vi "5.0.5_Inlet_Blockage_Calibration.vi"(6 "Data in":T1, 8 "error in (no error)":errorcluster, 9 "AllControls In":T2, 10 "?":T3, 11 "Message Queue out":T4) -> (0 "error out":errorcluster, 1 "Flow":string, 2 "Data":T3, 3 "Message Queue Out":T4, 4 "Data out":T1)   [LabVIEW 2017]
uses:
  Depends/AMC/subVIs/TypeDefs/amc_Message Queue.ctl
  Depends/AMC/subVIs/TypeDefs/amc_Message.ctl
  Depends/Tools/Keyed Array/Tools_KeyedArray KeyedArray.ctl
  Ctrls/Data.ctl
  Ctrls/AllControls.ctl
  Ctrls/CSV_Data.ctl
  DIPC 692 Daemon API/typdef/get_parameter.ctl
  DIPC 692 Daemon API/typdef/calibration.ctl
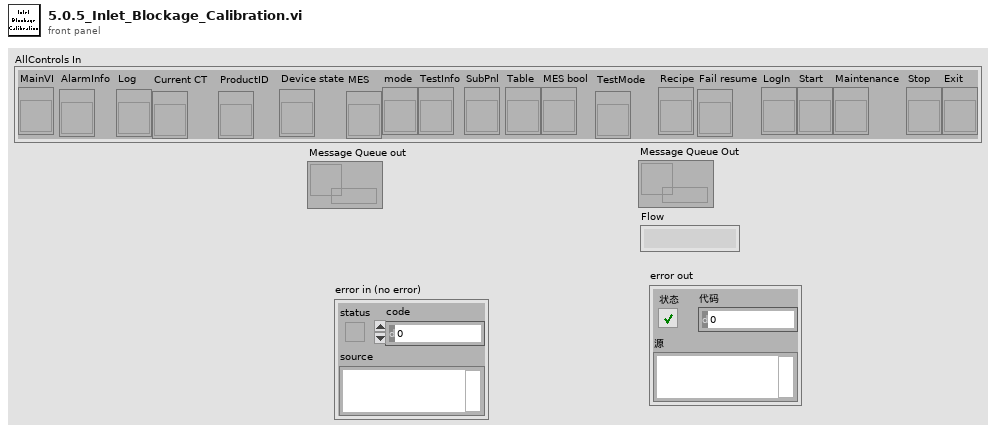
[diagram p1: front panel]
types:
  T1 = typedef "CSV_Data.ctl" = cluster{"Initialisation":cluster{"LMT - Connect UUT (con COM)":string, "LMT - Software Version (rrel)":string, "LMT - Write SKU file (wskuc)":string, "LMT - SKU file name":string, "Connect UUT DDM":string, "Read DDM EOL Timestamp - Mode":string, "Read DDM EOL Timestamp - Timestamp":string, "Read DDM EOL Timestamp - Rig ID":string, "Read DDM EOL Timestamp - Passmark ID":string, "Read DDM EOL Timestamp - Passmark Rev":string, "Software Version before flashing":string, "Read Hardware Serial":string, "UUT DDM SN":string, "Compare DDM SN with MES SN":string, "Backup PCBA Calibration EEPROM Response - CAL":string, "Flash Firmware Version":string, "Check SW Version":string, "Read DDM SW Version after flashing":string, "Set SKU Config":string, "Ready Status":string, "Set Device Mode to EOL":string, "DDM Parameter - Voltage":string, "DDM Parameter - Current":string, "DDM Parameter - Power":string, "DDM Parameter - Speed":string, "DDM Parameter - Pressure":string, "Tester Parameter - Voltage":string, "Tester Parameter - Current":string, "Tester Parameter - Power":string, "Tester Parameter - Ambient Pressure":string, "Tester Parameter - Ambient Temperature":string, "Calculated Parameter - DDM Pressure Corrected":string, "Calculated Parameter - DDM Real Power":string, "Calculated Parameter - Delta V":string}, "BEMF_Calibration":cluster{"Calibration Result - eol_cold_bemf_temp":string, "DDM Ambient Temp":string, "Restriction Plate Diameter":string, "Calibration Result - eol_bemf_mp_cold_coef_a":string, "Calibration Result - eol_bemf_mp_cold_coef_b":string, "Calibration Result - eol_bemf_mp_cold_coef_c":string, "Calibration Result - eol_bemf_lsi_cold_ref_coeffs":string, "Get - Calibration Result - eol_bemf_lsi_speed":string, "Get - Calibration Result - eol_bemf_lsi_integral_0":string, "Calibration Result - eol_bemf_lsi_integral_1":string, "Get - Calibration Result - eol_bemf_lsi_integral_2":string, "Get - Calibration Result - eol_cold_bemf":string, "Get - Calibration Result - eol_cold_bemf_fisf":string, "Finalise Calibration":string, "Compare -Calibration Result - eol_cold_bemf":string, "Compare -Calibration Result - eol_cold_bemf_fisf":string}, "ECO":cluster{"Reset Power Tune":string, "Reset BEMF FISF Calibration":string, "Restriction Plate Diameter":string, "ECO - Stabilisation Time":string, "ECO - DDM Parameter - Voltage":string, "ECO - DDM Parameter - Current":string, "ECO - DDM Parameter - Power":string, "ECO - DDM Parameter - Measured Power":string, "ECO - DDM Parameter - Speed":string, "ECO - DDM Parameter - Pressure":string, "ECO - Tester Parameter - Voltage":string, "ECO - Tester Parameter - Current":string, "ECO - Tester Parameter - Power":string, "ECO - Tester Parameter - Ambient Pressure":string, "ECO - Tester Parameter - Ambient Temperature":string, "ECO - Tester Parameter - Ambient Humidity":string, "ECO - Calculated Parameter - DDM Pressure Corrected":string, "ECO - Calculated Parameter - DDM Real Power":string, "ECO - Calculated Parameter - Delta V":string, "ECO - Calculated Parameter - Flowrate":string, "ECO - Calculated Parameter - Airwatt":string, "ECO - Formula":string, "PT ECO - Power Tune Mode Status":string}, "BOOST":cluster{"Restriction Plate Diameter":string, "BOOST - Stabilisation Time":string, "BOOST - DDM Parameter - Voltage":string, "BOOST - DDM Parameter - Current":string, "BOOST - DDM Parameter - Power":string, "BOOST - DDM Parameter - Measured Power":string, "BOOST - DDM Parameter - Speed":string, "BOOST - DDM Parameter - Pressure":string, "BOOST - Tester Parameter - Voltage":string, "BOOST - Tester Parameter - Current":string, "BOOST - Tester Parameter - Power":string, "BOOST - Tester Parameter - Ambient Pressure":string, "BOOST - Tester Parameter - Ambient Temperature":string, "BOOST - Tester Parameter - Ambient Humidity":string, "BOOST - Calculated Parameter - DDM Pressure Corrected":string, "BOOST - Calculated Parameter - DDM Real Power":string, "BOOST - Calculated Parameter - Delta V":string, "BOOST - Calculated Parameter - Flowrate":string, "BOOST - Calculated Parameter - Airwatt":string, "BOOST - Get AM Presence":string, "Air Muscle Turn Off Status":string, "BOOST - Air Muscle Calculated Parameter - Airwatt B":string, "BOOST - Air Muscle Calculate Airwatt Delta":string, "PT BOOST - Power Tune Mode Status":string, "Finalise Calibration":string, "ECO - Get AW Calibration value":string, "BOOST - Get AW Calibration value":string}, "MAX":cluster{"Restriction Plate Diameter":string, "MAX - Stabilisation Time":string, "Get Average Delta Tmag (LSIdelta_FISFdelta_LSItmag_FISFtmag_IIRtmag)":string, "Get Average Delta Tmag FISF":string, "MAX - DDM Parameter - Voltage":string, "MAX - DDM Parameter - Current":string, "MAX - DDM Parameter - Power":string, "MAX - DDM Parameter - Measured Power":string, "MAX - DDM Parameter - Speed":string, "MAX - DDM Parameter - Pressure":string, "MAX - Tester Parameter - Voltage":string, "MAX - Tester Parameter - Current":string, "MAX - Tester Parameter - Power":string, "MAX - Tester Parameter - Ambient Pressure":string, "MAX - Tester Parameter - Ambient Temperature":string, "MAX - Tester Parameter - Ambient Humidity":string, "MAX - Calculated Parameter - DDM Pressure Corrected":string, "MAX - Calculated Parameter - DDM Real Power":string, "MAX - Calculated Parameter - Delta V":string, "MAX - Calculated Parameter - Flowrate":string, "MAX - Calculated Parameter - Airwatt":string, "MAX_FISF_Check_Average_Delta_Tmag":string, "MAX - FISF - BEMF Finetune Result":string, "MAX tune - Delta P1":string, "MAX tune - Calculated Parameter - Airwatt":string, "Calculate Delta Airwatts - MAX finetune - Delta P2":string, "MAX finetune - DDM Parameter - Voltage":string, "MAX finetune - DDM Parameter - Current":string, "MAX finetune - DDM Parameter - Power":string, "MAX finetune - DDM Parameter - Measured Power":string, "MAX finetune - DDM Parameter - Speed":string, "MAX finetune - DDM Parameter - Pressure":string, "MAX finetune - Tester Parameter - Voltage":string, "MAX finetune - Tester Parameter - Current":string, "MAX finetune - Tester Parameter - Power":string, "MAX finetune - Tester Parameter - Ambient Pressure":string, "MAX finetune - Tester Parameter - Ambient Temperature":string, "MAX finetune - Tester Parameter - Ambient Humidity":string, "MAX finetune - Calculated Parameter - DDM Pressure Corrected":string, "MAX finetune - Calculated Parameter - DDM Real Power":string, "MAX finetune - Calculated Parameter - Delta V":string, "MAX finetune - Calculated Parameter - Flowrate":string, "MAX finetune - Calculated Parameter - Airwatt":string, "Check Derate Result":string, "Delta Tmag FISF":string, "Get Hot BEMF Result":string, "Calculate delta Pressure":string, "Finalise Calibration":string, "Calculate & Check Delta BEMF":string, "Delta P Airwatts Value":string}, "LL":cluster{"DDM Ambient Temp":string, "Restriction Plate Diameter":string, "LL - DDM Parameter - Voltage":string, "LL - DDM Parameter - Current":string, "LL - DDM Parameter - Power":string, "LL - DDM Parameter - Measured Power":string, "LL - DDM Parameter - Speed":string, "LL - DDM Parameter - Pressure":string, "LL - Tester Parameter - Voltage":string, "LL - Tester Parameter - Current":string, "LL - Tester Parameter - Power":string, "LL - DDM Real Power":string, "LL - Calibrate Task Detect LL":string}, "HL":cluster{"HL - DDM Parameter - Voltage":string, "HL - DDM Parameter - Current":string, "HL - DDM Parameter - Power":string, "HL - DDM Parameter - Measured Power":string, "HL - DDM Parameter - Speed":string, "HL - DDM Parameter - Pressure":string, "HL - Tester Parameter - Voltage":string, "HL - Tester Parameter - Current":string, "HL - Tester Parameter - Power":string, "HL - DDM Real Power":string, "HL - Calibrate Task Detect HL":string}, "LH":cluster{"Restriction Plate Diameter":string, "LH - DDM Parameter - Voltage":string, "LH - DDM Parameter - Current":string, "LH - DDM Parameter - Power":string, "LH - DDM Parameter - Measured Power":string, "LH - DDM Parameter - Speed":string, "LH - DDM Parameter - Pressure":string, "LH - Tester Parameter - Voltage":string, "LH - Tester Parameter - Current":string, "LH - Tester Parameter - Power":string, "LH - DDM Real Power":string, "LH - Calibrate Task Detect LH":string}, "HH":cluster{"HH - DDM Parameter - Voltage":string, "HH - DDM Parameter - Current":string, "HH - DDM Parameter - Power":string, "HH - DDM Parameter - Measured Power":string, "HH - DDM Parameter - Speed":string, "HH - DDM Parameter - Pressure":string, "HH - Tester Parameter - Voltage":string, "HH - Tester Parameter - Current":string, "HH - Tester Parameter - Power":string, "HH - DDM Real Power":string, "HH - Calibrate Task Detect HH":string}, "Inlet Blockage Calibration":cluster{"Inlet Blockage Calibration - DDM Parameter - Voltage":string, "Inlet Blockage Calibration - DDM Parameter - Current":string, "Inlet Blockage Calibration - DDM Parameter - Power":string, "Inlet Blockage Calibration - DDM Parameter - Measured Power":string, "Inlet Blockage Calibration - DDM Parameter - Speed":string, "Inlet Blockage Calibration - DDM Parameter - Pressure":string, "Inlet Blockage Calibration - Tester Parameter - Voltage":string, "Inlet Blockage Calibration - Tester Parameter - Current":string, "Inlet Blockage Calibration - Tester Parameter - Power":string, "Inlet Blockage Calibration - DDM Real Power":string, "Calibration Inlet Blockage_E":string, "Finalise Calibration":string, "Get Task Detect LL":string, "Get Task Detect HL":string, "Get Task Detect LH":string, "Get Task Detect HH":string, "Calibration Inlet Blockage":string, "Calibration eol cold bemf temp":string}, "GOOD":cluster{"GOOD UNIT - Clear EEPROM Error Log":string, "GOOD UNIT - Write Product Timestamp - Mode":string, "GOOD UNIT - Write Product Timestamp - Timestamp":string, "GOOD UNIT - Write Product Timestamp - Rig ID":string, "GOOD UNIT - Write Product Timestamp - Passmark ID":string, "GOOD UNIT - Write Product Timestamp - Passmark Rev":string, "GOOD UNIT - Set Device Mode to PROD":string, "GOOD UNIT - Backup PCBA Calibration EEPROM Response":string, "GOOD UNIT - Check Security Bit":string, "GOOD UNIT - Set Calibration Lock":string, "GOOD UNIT - Get_Calibration_Lock":string, "GOOD UNIT - Disconnect UUT":string}, "NG":cluster{"NG UNIT - Read NVM Error":string, "NG UNIT - Set Device Mode to FCT":string, "NG UNIT - Backup PCBA Calibration EEPROM Response - CAL":string, "NG UNIT - Backup PCBA Calibration EEPROM Response - ERROR":string, "NG UNIT - Backup PCBA Calibration EEPROM Response - USAGE":string, "NG UNIT - Disconnect UUT":string}, "SN":string, "Table":string[][], "Count":cluster{"Total":i32, "OK":i32, "NG":i32, "Yield":dbl}, "Start Time":timestamp, "daemon reference":refnum<k5>, "CT":dbl, "Config":string[][], "OK/NG":bool, "Station ID":string, "MES DDM SN":string, "MES PCBA SN":string, "Retest":string, "Lux":string, "Initialisation_Status":cluster{"LMT - Connect UUT (con COM)":string, "LMT - Software Version (rrel)":string, "LMT - Write SKU file (wskuc)":string, "LMT - SKU file name":string, "Connect UUT DDM":string, "Read DDM EOL Timestamp - Mode":string, "Read DDM EOL Timestamp - Timestamp":string, "Read DDM EOL Timestamp - Rig ID":string, "Read DDM EOL Timestamp - Passmark ID":string, "Read DDM EOL Timestamp - Passmark Rev":string, "Software Version before flashing":string, "Read Hardware Serial":string, "UUT DDM SN":string, "Compare DDM SN with MES SN":string, "Backup PCBA Calibration EEPROM Response - CAL":string, "Flash Firmware Version":string, "Check SW Version":string, "Read DDM SW Version after flashing":string, "Set SKU Config":string, "Ready Status":string, "Set Device Mode to EOL":string, "DDM Parameter - Voltage":string, "DDM Parameter - Current":string, "DDM Parameter - Power":string, "DDM Parameter - Speed":string, "DDM Parameter - Pressure":string, "Tester Parameter - Voltage":string, "Tester Parameter - Current":string, "Tester Parameter - Power":string, "Tester Parameter - Ambient Pressure":string, "Tester Parameter - Ambient Temperature":string, "Calculated Parameter - DDM Pressure Corrected":string, "Calculated Parameter - DDM Real Power":string, "Calculated Parameter - Delta V":string}, "BEMF_Calibration_Status":cluster{"Calibration Result - eol_cold_bemf_temp":string, "DDM Ambient Temp":string, "Restriction Plate Diameter":string, "Calibration Result - eol_bemf_mp_cold_coef_a":string, "Calibration Result - eol_bemf_mp_cold_coef_b":string, "Calibration Result - eol_bemf_mp_cold_coef_c":string, "Calibration Result - eol_bemf_lsi_cold_ref_coeffs":string, "Get - Calibration Result - eol_bemf_lsi_speed":string, "Get - Calibration Result - eol_bemf_lsi_integral_0":string, "Calibration Result - eol_bemf_lsi_integral_1":string, "Get - Calibration Result - eol_bemf_lsi_integral_2":string, "Get - Calibration Result - eol_cold_bemf":string, "Get - Calibration Result - eol_cold_bemf_fisf":string, "Finalise Calibration":string, "Compare -Calibration Result - eol_cold_bemf":string, "Compare -Calibration Result - eol_cold_bemf_fisf":string}, "ECO_Status":cluster{"Reset Power Tune":string, "Reset BEMF FISF Calibration":string, "Restriction Plate Diameter":string, "ECO - Stabilisation Time":string, "ECO - DDM Parameter - Voltage":string, "ECO - DDM Parameter - Current":string, "ECO - DDM Parameter - Power":string, "ECO - DDM Parameter - Measured Power":string, "ECO - DDM Parameter - Speed":string, "ECO - DDM Parameter - Pressure":string, "ECO - Tester Parameter - Voltage":string, "ECO - Tester Parameter - Current":string, "ECO - Tester Parameter - Power":string, "ECO - Tester Parameter - Ambient Pressure":string, "ECO - Tester Parameter - Ambient Temperature":string, "ECO - Tester Parameter - Ambient Humidity":string, "ECO - Calculated Parameter - DDM Pressure Corrected":string, "ECO - Calculated Parameter - DDM Real Power":string, "ECO - Calculated Parameter - Delta V":string, "ECO - Calculated Parameter - Flowrate":string, "ECO - Calculated Parameter - Airwatt":string, "ECO - Formula":string, "PT ECO - Power Tune Mode Status":string}, "BOOST_Status":cluster{"Restriction Plate Diameter":string, "BOOST - Stabilisation Time":string, "BOOST - DDM Parameter - Voltage":string, "BOOST - DDM Parameter - Current":string, "BOOST - DDM Parameter - Power":string, "BOOST - DDM Parameter - Measured Power":string, "BOOST - DDM Parameter - Speed":string, "BOOST - DDM Parameter - Pressure":string, "BOOST - Tester Parameter - Voltage":string, "BOOST - Tester Parameter - Current":string, "BOOST - Tester Parameter - Power":string, "BOOST - Tester Parameter - Ambient Pressure":string, "BOOST - Tester Parameter - Ambient Temperature":string, "BOOST - Tester Parameter - Ambient Humidity":string, "BOOST - Calculated Parameter - DDM Pressure Corrected":string, "BOOST - Calculated Parameter - DDM Real Power":string, "BOOST - Calculated Parameter - Delta V":string, "BOOST - Calculated Parameter - Flowrate":string, "BOOST - Calculated Parameter - Airwatt":string, "BOOST - Get AM Presence":string, "Air Muscle Turn Off Status":string, "BOOST - Air Muscle Calculated Parameter - Airwatt B":string, "BOOST - Air Muscle Calculate Airwatt Delta":string, "PT BOOST - Power Tune Mode Status":string, "Finalise Calibration":string, "ECO - Get AW Calibration value":string, "BOOST - Get AW Calibration value":string}, "MAX_Status":cluster{"Restriction Plate Diameter":string, "MAX - Stabilisation Time":string, "Get Average Delta Tmag (LSIdelta_FISFdelta_LSItmag_FISFtmag_IIRtmag)":string, "Get Average Delta Tmag FISF":string, "MAX - DDM Parameter - Voltage":string, "MAX - DDM Parameter - Current":string, "MAX - DDM Parameter - Power":string, "MAX - DDM Parameter - Measured Power":string, "MAX - DDM Parameter - Speed":string, "MAX - DDM Parameter - Pressure":string, "MAX - Tester Parameter - Voltage":string, "MAX - Tester Parameter - Current":string, "MAX - Tester Parameter - Power":string, "MAX - Tester Parameter - Ambient Pressure":string, "MAX - Tester Parameter - Ambient Temperature":string, "MAX - Tester Parameter - Ambient Humidity":string, "MAX - Calculated Parameter - DDM Pressure Corrected":string, "MAX - Calculated Parameter - DDM Real Power":string, "MAX - Calculated Parameter - Delta V":string, "MAX - Calculated Parameter - Flowrate":string, "MAX - Calculated Parameter - Airwatt":string, "MAX_FISF_Check_Average_Delta_Tmag":string, "MAX - FISF - BEMF Finetune Result":string, "MAX tune - Delta P1":string, "MAX tune - Calculated Parameter - Airwatt":string, "Calculate Delta Airwatts - MAX finetune - Delta P2":string, "MAX finetune - DDM Parameter - Voltage":string, "MAX finetune - DDM Parameter - Current":string, "MAX finetune - DDM Parameter - Power":string, "MAX finetune - DDM Parameter - Measured Power":string, "MAX finetune - DDM Parameter - Speed":string, "MAX finetune - DDM Parameter - Pressure":string, "MAX finetune - Tester Parameter - Voltage":string, "MAX finetune - Tester Parameter - Current":string, "MAX finetune - Tester Parameter - Power":string, "MAX finetune - Tester Parameter - Ambient Pressure":string, "MAX finetune - Tester Parameter - Ambient Temperature":string, "MAX finetune - Tester Parameter - Ambient Humidity":string, "MAX finetune - Calculated Parameter - DDM Pressure Corrected":string, "MAX finetune - Calculated Parameter - DDM Real Power":string, "MAX finetune - Calculated Parameter - Delta V":string, "MAX finetune - Calculated Parameter - Flowrate":string, "MAX finetune - Calculated Parameter - Airwatt":string, "Check Derate Result":string, "Delta Tmag FISF":string, "Get Hot BEMF Result":string, "Calculate delta Pressure":string, "Finalise Calibration":string, "Calculate & Check Delta BEMF":string, "Delta P Airwatts Value":string}, "LL_Status":cluster{"DDM Ambient Temp":string, "Restriction Plate Diameter":string, "LL - DDM Parameter - Voltage":string, "LL - DDM Parameter - Current":string, "LL - DDM Parameter - Power":string, "LL - DDM Parameter - Measured Power":string, "LL - DDM Parameter - Speed":string, "LL - DDM Parameter - Pressure":string, "LL - Tester Parameter - Voltage":string, "LL - Tester Parameter - Current":string, "LL - Tester Parameter - Power":string, "LL - DDM Real Power":string, "LL - Calibrate Task Detect LL":string}, "HL_Status":cluster{"HL - DDM Parameter - Voltage":string, "HL - DDM Parameter - Current":string, "HL - DDM Parameter - Power":string, "HL - DDM Parameter - Measured Power":string, "HL - DDM Parameter - Speed":string, "HL - DDM Parameter - Pressure":string, "HL - Tester Parameter - Voltage":string, "HL - Tester Parameter - Current":string, "HL - Tester Parameter - Power":string, "HL - DDM Real Power":string, "HL - Calibrate Task Detect HL":string}, "LH_Status":cluster{"Restriction Plate Diameter":string, "LH - DDM Parameter - Voltage":string, "LH - DDM Parameter - Current":string, "LH - DDM Parameter - Power":string, "LH - DDM Parameter - Measured Power":string, "LH - DDM Parameter - Speed":string, "LH - DDM Parameter - Pressure":string, "LH - Tester Parameter - Voltage":string, "LH - Tester Parameter - Current":string, "LH - Tester Parameter - Power":string, "LH - DDM Real Power":string, "LH - Calibrate Task Detect LH":string}, "HH_Status":cluster{"HH - DDM Parameter - Voltage":string, "HH - DDM Parameter - Current":string, "HH - DDM Parameter - Power":string, "HH - DDM Parameter - Measured Power":string, "HH - DDM Parameter - Speed":string, "HH - DDM Parameter - Pressure":string, "HH - Tester Parameter - Voltage":string, "HH - Tester Parameter - Current":string, "HH - Tester Parameter - Power":string, "HH - DDM Real Power":string, "HH - Calibrate Task Detect HH":string}, "Inlet Blockage Calibration_Status":cluster{"Inlet Blockage Calibration - DDM Parameter - Voltage":string, "Inlet Blockage Calibration - DDM Parameter - Current":string, "Inlet Blockage Calibration - DDM Parameter - Power":string, "Inlet Blockage Calibration - DDM Parameter - Measured Power":string, "Inlet Blockage Calibration - DDM Parameter - Speed":string, "Inlet Blockage Calibration - DDM Parameter - Pressure":string, "Inlet Blockage Calibration - Tester Parameter - Voltage":string, "Inlet Blockage Calibration - Tester Parameter - Current":string, "Inlet Blockage Calibration - Tester Parameter - Power":string, "Inlet Blockage Calibration - DDM Real Power":string, "Calibration Inlet Blockage_E":string, "Finalise Calibration":string, "Get Task Detect LL":string, "Get Task Detect HL":string, "Get Task Detect LH":string, "Get Task Detect HH":string, "Calibration Inlet Blockage":string, "Calibration eol cold bemf temp":string}, "GOOD_Status":cluster{"GOOD UNIT - Clear EEPROM Error Log":string, "GOOD UNIT - Write Product Timestamp - Mode":string, "GOOD UNIT - Write Product Timestamp - Timestamp":string, "GOOD UNIT - Write Product Timestamp - Rig ID":string, "GOOD UNIT - Write Product Timestamp - Passmark ID":string, "GOOD UNIT - Write Product Timestamp - Passmark Rev":string, "GOOD UNIT - Set Device Mode to PROD":string, "GOOD UNIT - Backup PCBA Calibration EEPROM Response":string, "GOOD UNIT - Check Security Bit":string, "GOOD UNIT - Set Calibration Lock":string, "GOOD UNIT - Get_Calibration_Lock":string, "GOOD UNIT - Disconnect UUT":string}, "NG_Status":cluster{"NG UNIT - Read NVM Error":string, "NG UNIT - Set Device Mode to FCT":string, "NG UNIT - Backup PCBA Calibration EEPROM Response - CAL":string, "NG UNIT - Backup PCBA Calibration EEPROM Response - ERROR":string, "NG UNIT - Backup PCBA Calibration EEPROM Response - USAGE":string, "NG UNIT - Disconnect UUT":string}, "SKU":string, "Plate_Diameter":string, "Alarm":string}
  T2 = typedef "AllControls.ctl" = cluster{"MainVI":refnum<vi>, "AlarmInfo":refnum<vi>, "Log":refnum<vi>, "Current CT":refnum<vi>, "ProductID":refnum<vi>, "Device state":refnum<vi>, "MES":refnum<vi>, "mode":refnum<vi>, "TestInfo":refnum<vi>, "SubPnl":refnum<vi>, "Table":refnum<vi>, "MES bool":refnum<vi>, "TestMode":refnum<vi>, "Recipe":refnum<vi>, "Fail resume":refnum<vi>, "LogIn":refnum<vi>, "Start":refnum<vi>, "Maintenance":refnum<vi>, "Stop":refnum<vi>, "Exit":refnum<vi>}
  T3 = typedef "Data.ctl" = cluster{"Initialisation":cluster{"DDM_Parameter":dbl[], "DDM_Parameter_status":bool[], "Get_Tester_Parameter":dbl[], "Get_Tester_Parameter_status":bool[], "Cal_Tester_Parameter":dbl[], "Cal_Tester_Parameter_status":bool[], "sw_version_before_status":bool, "sw_version_after_status":bool, "Set_SKU_Config_With_LMT_status":bool, "FCT_timestamp_status":bool, "LMT_Connect_to_UUT_status":bool}, "BEMF_Calibration":cluster{"Read_ambient_temperature":dbl, "Calibration_Vaule":dbl[], "Calibration_Vaule _B":dbl[], "Calibration_Vaule_status":bool[], "Calibration_Vaule_B_status":bool[]}, "ECO":cluster{"DDM_Parameter":dbl[], "DDM_Parameter_status":bool[], "Get_Tester_Parameter":dbl[], "Get_Tester_Parameter_status":bool[], "Cal_Tester_Parameter":dbl[], "Cal_Tester_Parameter_status":bool[], "DDM_Parameter_after_power_tune":dbl[], "Get_Tester_Parameter_after_power_tune":dbl[], "Cal_Tester_Parameter_after_power_tune":dbl[], "Cal_Tester_Parameter_after_power_tune_status":bool[], "Delta_P":dbl}, "BOOST":cluster{"DDM_Parameter":dbl[], "DDM_Parameter_status":bool[], "Get_Tester_Parameter":dbl[], "Get_Tester_Parameter_status":bool[], "Cal_Tester_Parameter":dbl[], "Cal_Tester_Parameter_status":bool[], "DDM_Parameter_after_power_tune":dbl[], "Get_Tester_Parameter_after_power_tune":dbl[], "Cal_Tester_Parameter_after_power_tune":dbl[], "Cal_Tester_Parameter_after_power_tune_status":bool[], "airwatts_am_off":dbl, "AW_Delta_(AM_on_and_off)":dbl, "AW_Delta_(AM_on_and_off)_Status":bool, "Delta_P":dbl}, "MAX":cluster{"Average_Tmag_Data":cluster{"LSI Delta in degC":dbl, "FISF Delta in degc":dbl, "LSI Tmag in degC":dbl, "Fisf Tmag in degC":dbl, "IIR Tmag in degC":dbl}, "DDM_Parameter":dbl[], "DDM_Parameter_status":bool[], "Get_Tester_Parameter":dbl[], "Get_Tester_Parameter_status":bool[], "Cal_Tester_Parameter":dbl[], "BEMF_Finetune":cluster{"eol_bemf_mp_cold_coef_c":dbl, "eol_cold_bemf_fisf_offset":dbl}, "AW_Tune":cluster{"delta_P1":dbl, "delta_P_Setting":dbl}, "DDM_Parameter_after_Airwatts_Tune":dbl[], "Get_Tester_Parameter_after_Airwatts_Tune":dbl[], "Cal_Tester_Parameter_after_Airwatts_Tune":dbl[], "DDM_Parameter_after_Airwatts_Finetune":dbl[], "Get_Tester_Parameter_after_Airwatts_Finetune":dbl[], "Cal_Tester_Parameter_after_Airwatts_Finetune":dbl[], "AW_Finetune":cluster{"delta_P2":dbl, "delta_P_Setting":dbl}, "Delta_Tmag_after_tune":cluster{"LSI Delta in degC":dbl, "FISF Delta in degc":dbl, "LSI Tmag in degC":dbl, "Fisf Tmag in degC":dbl, "IIR Tmag in degC":dbl}, "Hot Bemf in mV":dbl, "DDM_Pressure":dbl, "Delta_Pressure":dbl, " Cold Bemf in mV":dbl, " delta Bemf":dbl, " delta p":dbl, "Delta_Pressure_status":bool, " delta Bemf_status":bool, "LSI Delta in degC_status":bool, "FISF Delta in degc_status":bool, "Max_check_derate_status_status":bool, "Average_All_data":dbl[][], "Average_Tmag_Data_status":bool[], "Average_Tmag_Data_after_tune_status":bool[], "Cal_Tester_Parameter_status":bool[], "Cal_Tester_Parameter_status_after_Airwatts_Tune":bool[], "Cal_Tester_Parameter_status_after_Airwatts_FineTune":bool[]}, "Task_Detect_Calib":cluster{"LL":cluster{"DDM_Parameter":dbl[], "DDM_Parameter_status":bool[], "Get_Tester_Parameter":dbl[], "Get_Tester_Parameter_status":bool[], "Set_task_detect_A":dbl, "Set_task_detect_A_Status":bool}, "HL":cluster{"DDM_Parameter":dbl[], "DDM_Parameter_status":bool[], "Get_Tester_Parameter":dbl[], "Get_Tester_Parameter_status":bool[], "Set_task_detect_B":dbl, "Set_task_detect_B_Status":bool}, "LH":cluster{"DDM_Parameter":dbl[], "DDM_Parameter_status":bool[], "Get_Tester_Parameter":dbl[], "Get_Tester_Parameter_status":bool[], "Set_task_detect_C":dbl, "Set_task_detect_C_Status":bool}, "HH":cluster{"DDM_Parameter":dbl[], "DDM_Parameter_status":bool[], "Get_Tester_Parameter":dbl[], "Get_Tester_Parameter_status":bool[], "Set_task_detect_D":dbl, "Read_and_check_calibration_Status":bool[], "Set_task_detect_D_Status":bool}, "Get_eol_inlet_blockage_E":dbl, "Calib_vaule":cluster{"Get_task_detect_LL":dbl, "Get_task_detect_HL":dbl, "Get_task_detect_LH":dbl, "Get_task_detect_HH":dbl, "eol_inlet_blockage":dbl, "eol_code_bemf_temp":dbl}, "calibrated temp":dbl, "Inlet_Blockage_Calibration":cluster{"DDM_Parameter":dbl[], "DDM_Parameter_status":bool[], "Get_Tester_Parameter":dbl[], "Get_Tester_Parameter_status":bool[]}, "Get_eol_inlet_blockage_E_Status":bool}, "good":cluster{"Write_Product_TS":cluster{"TIMESTAMP":i64, "RIG_ID":i64, "PASSMARK_ID":i64, "PASSMARK_REV":i64}, "Read_Product_TS":cluster{"TIMESTAMP":i64, "RIG_ID":i64, "PASSMARK_ID":i64, "PASSMARK_REV":i64}, "Good_Check_Secuity_Bit_Stauts":bool}}
  T4 = typedef "amc_Message Queue.ctl" = refnum<queue>
  T5 = typedef "HD Config.ctl" = cluster{" PC":cluster{"PC Address":u8[], "PC Port":i32}, "FCO":cluster{"COM":refnum<visa-resource-name>, "Baudrate":u32}, "DC Power ":cluster{"COM":refnum<visa-resource-name>, "Baudrate":u32}, "PW3336":cluster{"COM":refnum<visa-resource-name>, "Baudrate":u32}, "Lefoo":cluster{"COM":refnum<visa-resource-name>, "Baudrate":u32}, "Tempt&Hum":cluster{"COM":refnum<visa-resource-name>, "Baudrate":u32}, "DIPC":cluster{"COM":refnum<visa-resource-name>}, "Daemon":cluster{"IP Address":string, "Port":u16, "Retry":u16}, "URAT":cluster{"COM":refnum<visa-resource-name>, "Baudrate":u32}, "Fail_resume_mode":bool, "GRR":bool}
  T6 = typedef "get_parameter.ctl" = string
  T7 = typedef "calibration.ctl" = string
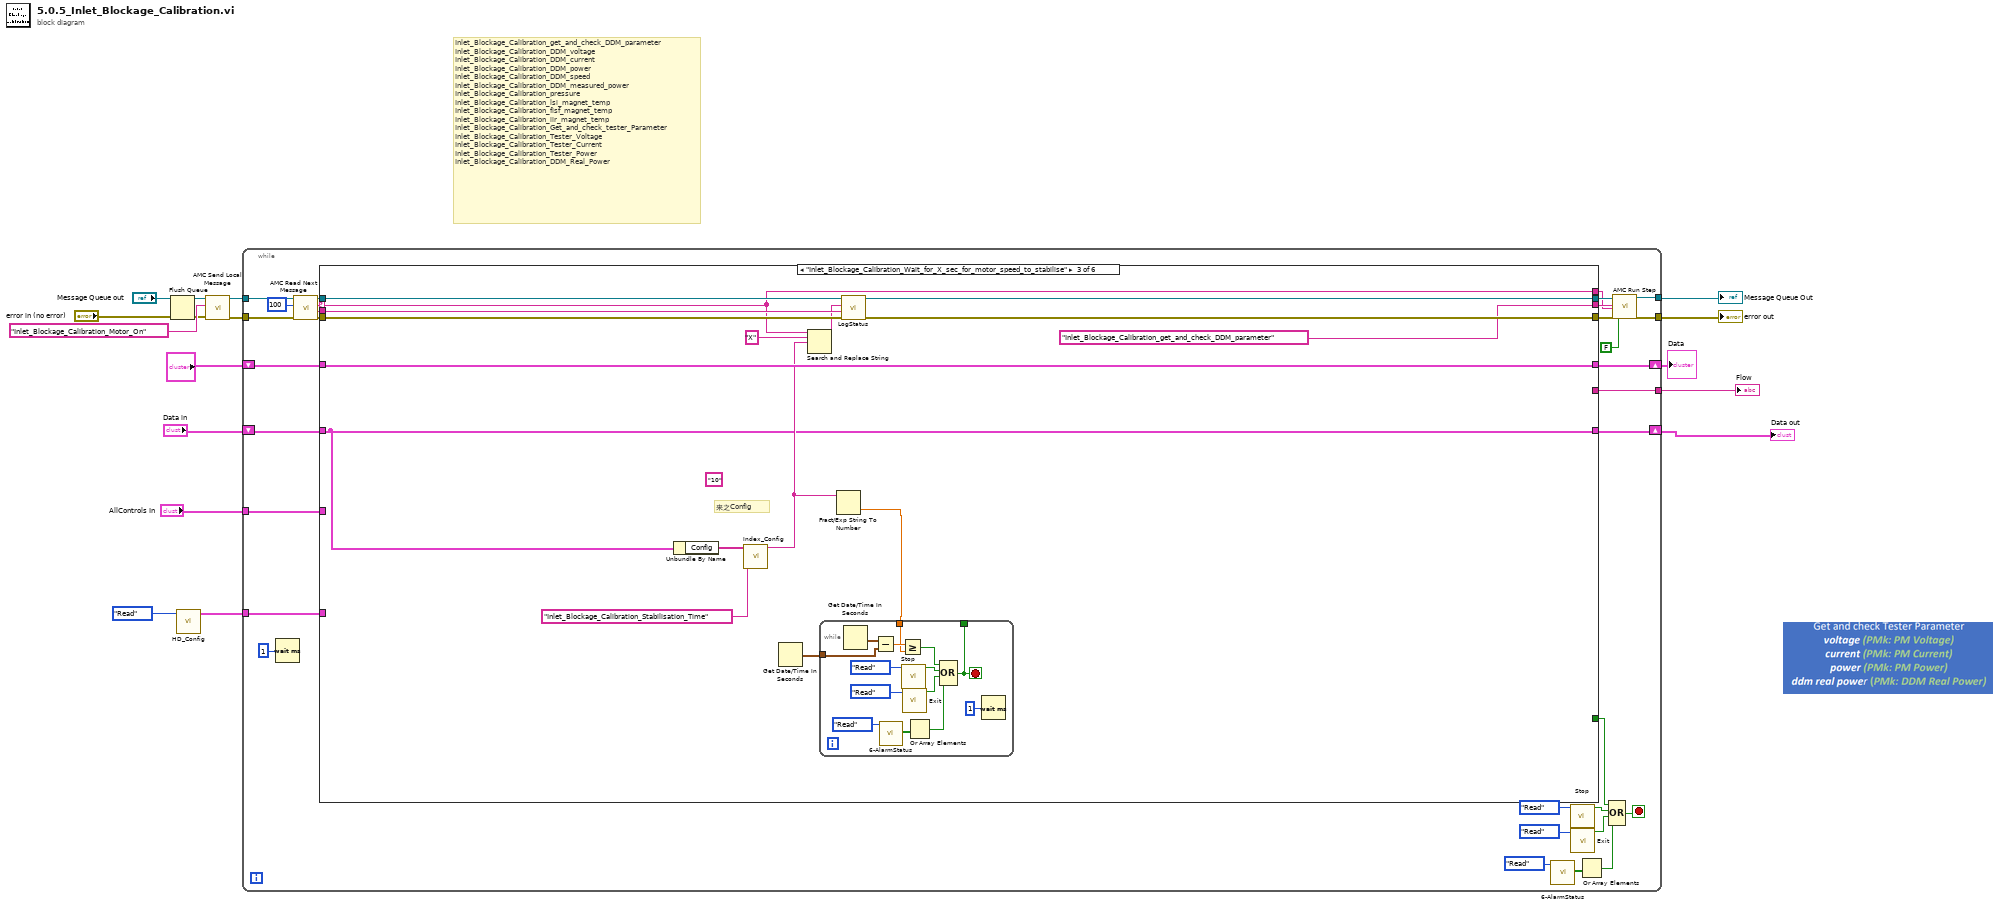
[diagram p0: block diagram]
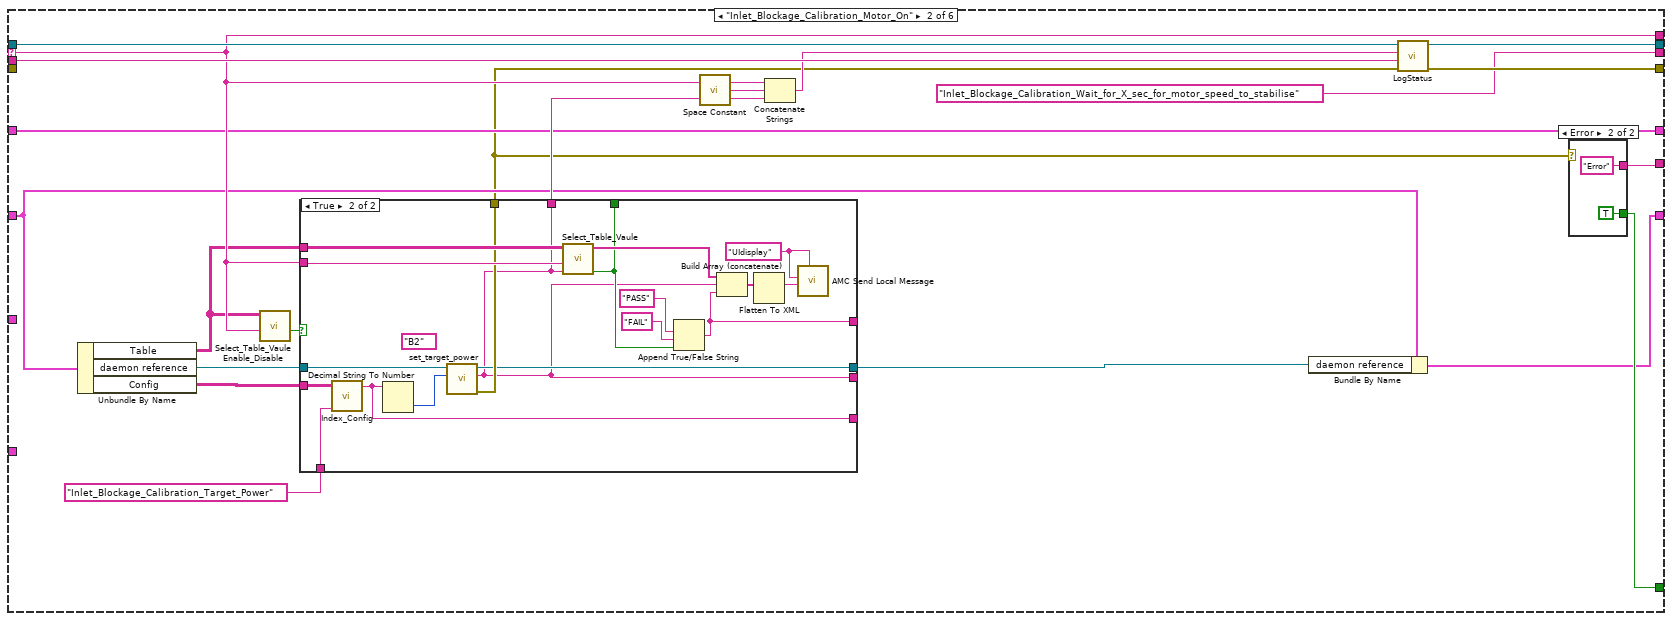
[diagram p3: hidden frame]
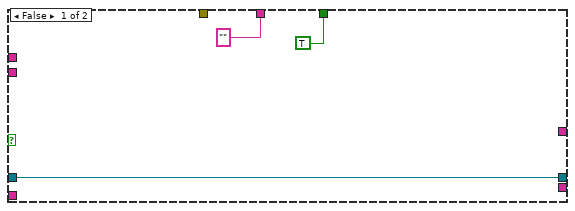
[diagram p5: hidden frame]
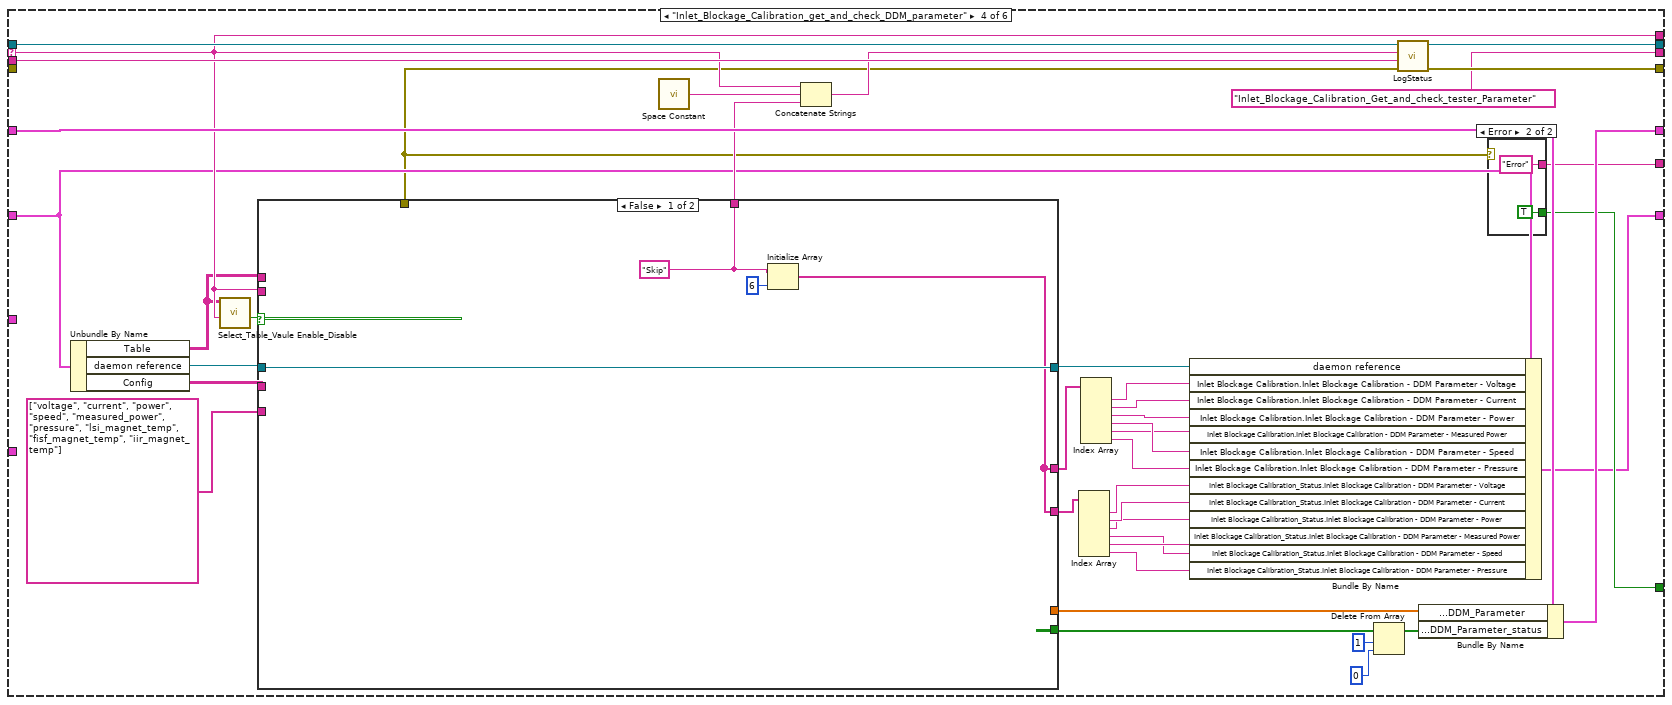
[diagram p6: hidden frame]
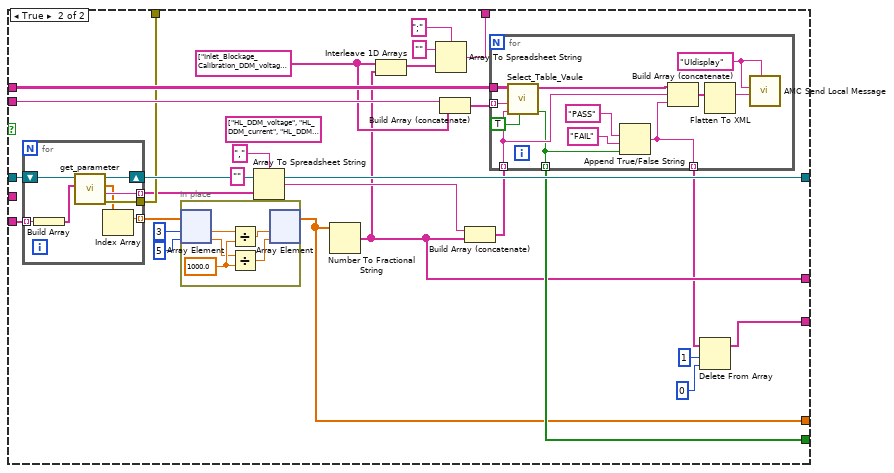
[diagram p8: hidden frame]
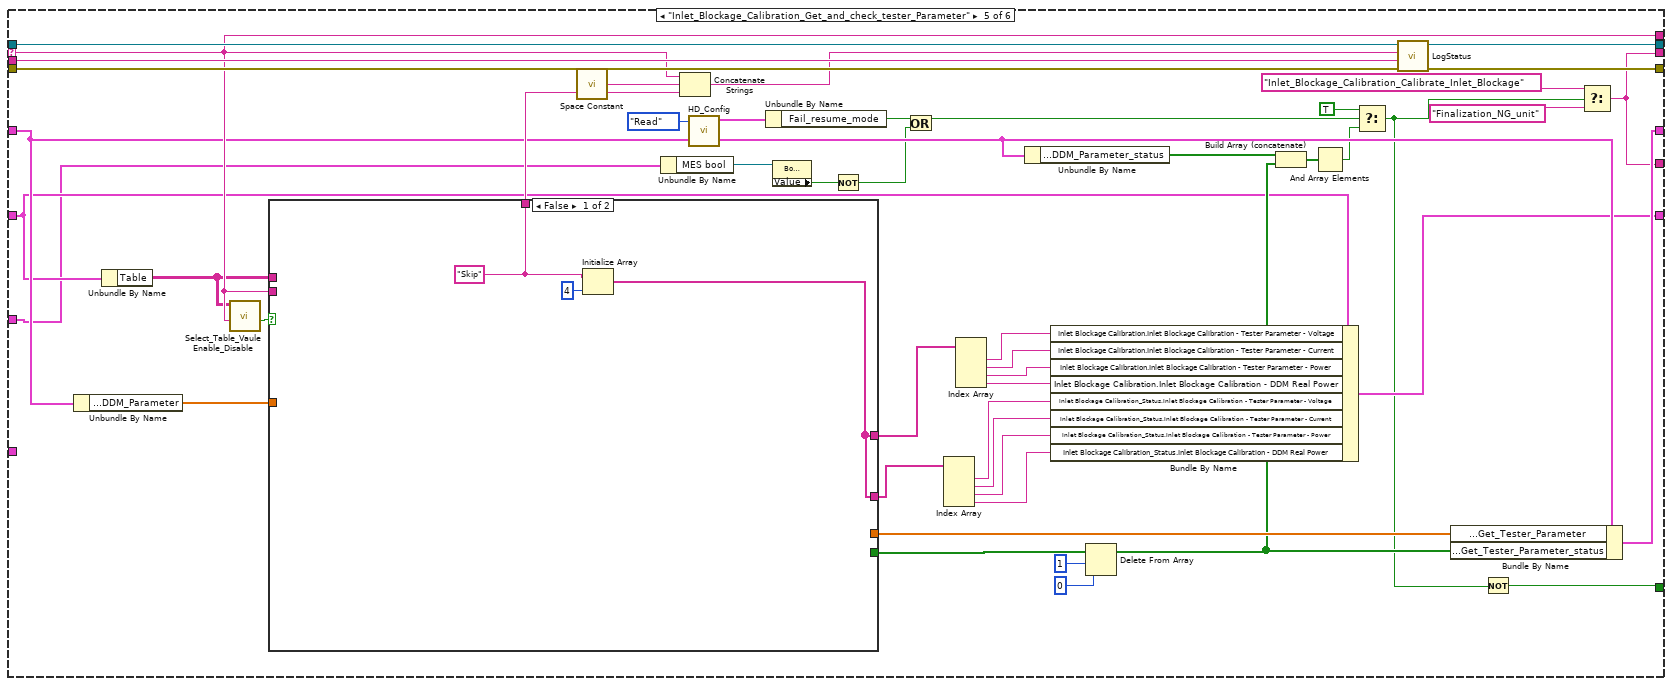
[diagram p9: hidden frame]
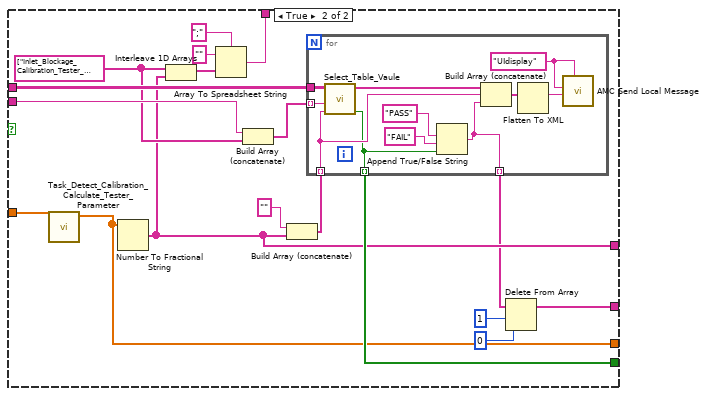
[diagram p10: hidden frame]
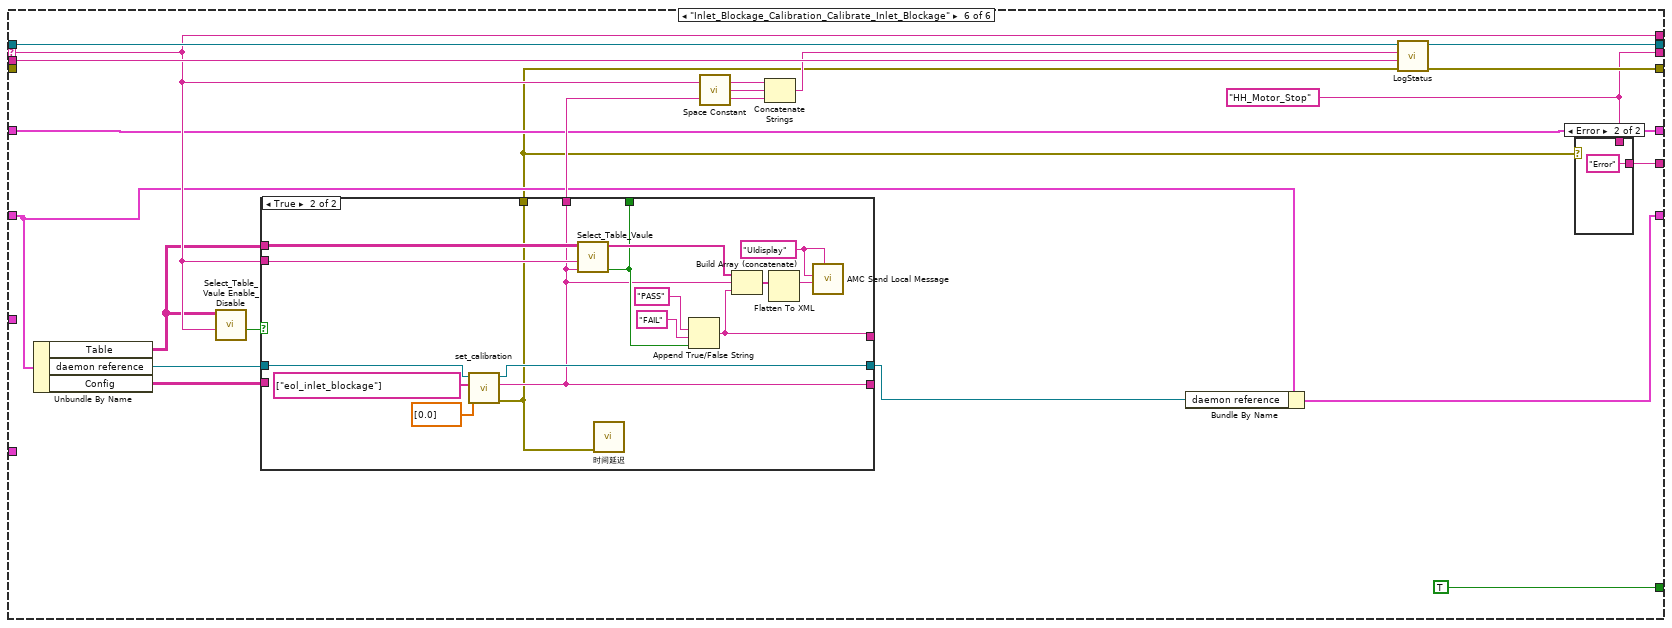
[diagram p11: hidden frame]
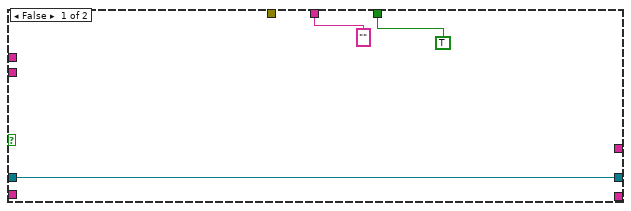
[diagram p13: hidden frame]
diagram:
  # "Inlet_Blockage_Calibration_get_and_check_DDM_parameter\nInlet_Blockage_Calibration_DDM_voltage\nInlet_Blockage_Calibration_DDM_current\nInlet_Blockage_Calibration_DDM_power\nInlet_Blockage_Calibration_DDM_speed\nInlet_Blockage_Calibration_DDM_measured_power\nInlet_Blockage_Calibration_pressure\nInlet_Blockage_Calibration_lsi_magnet_temp\nInlet_Blockage_Calibration_fisf_magnet_temp\nInlet_Blockage_Calibration_iir_magnet_temp\nInlet_Blockage_Calibration_Get_and_check_tester_Parameter\nInlet_Blockage_Calibration_Tester_Voltage\nInlet_Blockage_Calibration_Tester_Current\nInlet_Blockage_Calibration_Tester_Power\nInlet_Blockage_Calibration_DDM_Real_Power"
  n1 = Flush Queue(queue="Message Queue out") -> (queue out=w4:T4)  [unwired: 1 in, 2 out]
  n2 = call "HD_Config.vi"("Step"=enum16{"Initial", "Write", "Read"}."Read") -> ("HD Config out"=w8:T5)  [unwired: 9 in, 1 out]
  n3 = call "AMC Send Local Message.vi"("error in (no error)"="error in (no error)", "Message Name"="Inlet_Blockage_Calibration_Motor_On", "Message Queue in"=w4) -> ("error out"=w13:errorcluster, "Message Queue out"=w14:T4)  [unwired: 7 in]
  n4 = while {
    tunnel: w14 -> [w47]
    tunnel: [w43] -> w6
    tunnel: w13 -> [w41]
    tunnel: [w38] -> w5
    shift-right: [w34] -> w10
    shift-left: "?" -> [w35]
    tunnel: w8 -> [w33]
    tunnel: [w29] -> w7
    shift-right: [w20] -> w1
    shift-left: "Data in" -> [w22]
    tunnel: "AllControls In" -> [w21]
    stop <- w23 stop-if-true
    n5 = Wait (ms)(milliseconds to wait=u32 1 ("等待时间（毫秒）")) -> ()  [unwired: 1 out]
    n6 = call "AMC Read Next Message.vi"("error in (no error)"=w41, "timeout (1ms)"=100, "Message Queue in"=w47) -> ("error out"=w40:errorcluster, "Message Value"=w31:string, "Message Name"=w45:string, "Message Queue out"=w46:T4)  [unwired: 1 in, 4 out]
    n7 = case shown="\"Inlet_Blockage_Calibration_Wait_for_X_sec_for_motor_speed_to_stabilise\"" w45 {
      selector: w45 -> [_ w64 w103 w154 w260 w311]
      tunnel: w46 -> [w51 w71 w109 w163 w268 w319]
      tunnel: [w51 w71 w109 w163 w268 w319] -> w44
      tunnel: w40 -> [w50 _ w108 _ w267 _]
      tunnel: [w50 w70 w107 w162 w266 w318] -> w39
      tunnel: [_ w58 _ w144 w252 TRUE] -> w24
      tunnel: w35 -> [w49 w56 w101 w159 w255 w305]
      tunnel: [w49 w56 w101 w158 w264 w305] -> w34
      tunnel: w31 -> [_ w69 w106 w161 w265 w317]
      tunnel: [_ w64 w103 w154 w260 w311] -> w30
      tunnel: w33 -> [_ _ _ _ _ _]
      tunnel: [_ "Inlet_Blockage_Calibration_Wait_for_X_sec_for_motor_speed_to_stabilise" "Inlet_Blockage_Calibration_get_and_check_DDM_parameter" "Inlet_Blockage_Calibration_Get_and_check_tester_Parameter" w251 w307] -> w32
      tunnel: [_ w59 _ w143 w251 w308] -> w29
      tunnel: w22 -> [w48 w55 w95 w141 w244 w304]
      tunnel: w21 -> [_ _ _ _ w233 _]
      tunnel: [w48 w54 w95 w137 w242 w303] -> w20
      frame "假", Default {
      }
      frame "Inlet_Blockage_Calibration_Motor_On" {
        n8 = Unbundle By Name(w55) -> ("Table"=w63:string[][], "daemon reference"=w68:refnum<k5>, "Config"=w61:string[][])
        n9 = call "Select_Table_Vaule Enable_Disable.vi"("Action"=w64, "Table"=w63) -> ("Enable"=w65:bool)  [unwired: 8 in, 1 out]
        n10 = case shown="True" w65 {
          tunnel: w68 -> [w75 w83]
          tunnel: [TRUE w86] -> _
          tunnel: [w75 w81] -> w53
          tunnel: ["" ("response") w77] -> w57
          tunnel: w64 -> [_ w89]
          tunnel: w63 -> [_ w88]
          tunnel: w61 -> [_ w85]
          tunnel: "Inlet_Blockage_Calibration_Target_Power" -> [_ w84]
          tunnel: [_ w82] -> w52
          tunnel: [_ w79] -> _
          tunnel: [_ w78] -> _
          tunnel: [_ w77] -> _
          frame False {
          }
          frame True {
            (unwired) "B2" ("Power Mode")
            w94 = "UIdisplay" ("Process (\"\" - local)")
            n11 = call "Index_Config.vi"("Action"=w84, "config"=w85) -> ("data"=w79:string)  [unwired: 9 in]
            n12 = Decimal String To Number(string=w79) -> (number=w80:i32)  [unwired: 2 in, 1 out]
            n13 = call "set_target_power.vi"("Power mW"=w80, "daemon reference in"=w83) -> ("error out"=w82:errorcluster, "response"=w77:string, "daemon reference out"=w81:refnum<k5>)  [unwired: 6 in, 1 out]
            n14 = call "Select_Table_Vaule.vi"("Vaule"=w77, "Action"=w89, "Table"=w88) -> ("Result"=w86:bool, "vaule"=w87:string[])  [unwired: 7 in]
            n15 = Append True/False String(1:w86, 2:"FAIL" ("真字符串"), 3:"PASS" ("真字符串")) -> (0:w78:string)  [unwired: 1 in]
            n16 = Build Array (concatenate)(w87, w77, w78) -> (w93:string[])
            n17 = Flatten To XML(anything=w93) -> (xml string=w92:string)
            n18 = call "AMC Send Local Message.vi"("Process (\"\" - local)"=w94, "Message Value"=w92, "Message Name"=w94) -> ()  [unwired: 7 in, 2 out]
          }
        }
        n19 = call <vilib>:"Space Constant.vi"() -> ("String"=w67:string)
        n20 = Concatenate Strings(w64, w67, w57) -> (w66:string)
        n21 = Bundle By Name(cluster=w55, "daemon reference"=w53) -> (w54:T1)
        n22 = call "LogStatus.vi"("error in (no error)"=w52, "last message"=w69, "message"=w66) -> ("error  out"=w70:errorcluster)  [unwired: 8 in]
        n23 = case shown="Error" w52 {
          tunnel: [_ TRUE] -> w58
          tunnel: [_ "Error"] -> w59
          frame No Error {
          }
          frame Error {
          }
        }
      }
      frame "Inlet_Blockage_Calibration_Wait_for_X_sec_for_motor_speed_to_stabilise" {
        (unwired) "10" ("替换字符串(\"\")")
        # "来之Config"
        n24 = Unbundle By Name(w95) -> ("Config"=w100:string[][])
        n25 = call "Index_Config.vi"("Action"="Inlet_Blockage_Calibration_Stabilisation_Time" ("替换字符串(\"\")"), "config"=w100) -> ("data"=w98:string)  [unwired: 9 in]
        n26 = Get Date/Time In Seconds() -> (seconds since 1Jan1904=w97:timestamp)
        n27 = Search and Replace String(input string=w103, search string="X" ("搜索字符串"), replace string=w98) -> (result string=w104:string)  [unwired: 5 in, 3 out]
        n28 = Fract/Exp String To Number(string=w98) -> (number=w96:dbl)  [unwired: 3 in, 1 out]
        n29 = while {
          tunnel: w97 -> [w116]
          tunnel: w96 -> [w113]
          tunnel: [w112] -> _
          stop <- w112 stop-if-true
          n30 = Get Date/Time In Seconds() -> (seconds since 1Jan1904=w117:timestamp)
          n31 = Subtract(x=w117, y=w116) -> (x-y=w115:dbl)
          n32 = call "6-AlarmStatus.vi"("Step"=enum16{"Initial", "Write", "Read"}."Read") -> ("AlarmValue Out"=w120:bool[])  [unwired: 9 in, 1 out]
          n33 = Greater Or Equal?(x=w115, y=w113) -> (x >= y?=w114:bool)
          n34 = call "Stop.vi"("Step"=enum16{"Initial", "Write", "Read"}."Read") -> ("Stop Out"=w118:bool)  [unwired: 9 in, 1 out]
          n35 = call "Exit.vi"("Step"=enum16{"Initial", "Write", "Read"}."Read" ("step")) -> ("Exit Out"=w122:bool)  [unwired: 9 in, 1 out]
          n36 = Or Array Elements(Boolean array=w120) -> (logical OR=w119:bool)
          n37 = Compound Arithmetic op=OR(w114, w118, w122, w119) -> (w112:bool)
          n38 = Wait (ms)(milliseconds to wait=u32 1 ("等待时间（毫秒）")) -> ()  [unwired: 1 out]
        }
        n39 = call "LogStatus.vi"("error in (no error)"=w108, "last message"=w106, "message"=w104) -> ("error  out"=w107:errorcluster)  [unwired: 8 in]
      }
      frame "Inlet_Blockage_Calibration_get_and_check_DDM_parameter" {
        n40 = Unbundle By Name(w141) -> ("Table"=w153:string[][], "daemon reference"=w160:refnum<k5>, "Config"=w151:string[][])
        n41 = call "Select_Table_Vaule Enable_Disable.vi"("Action"=w154, "Table"=w153) -> ("Enable"=w152:bool)  [unwired: 8 in, 1 out]
        n42 = case shown="False" w152 {
          tunnel: w160 -> [w169 w195]
          tunnel: [w169 w194] -> w138
          tunnel: [w166 w186] -> w155
          tunnel: w154 -> [_ w191]
          tunnel: w153 -> [_ w196]
          tunnel: w151 -> [_ _]
          tunnel: [_ w181] -> w149
          tunnel: [_ w193] -> w148
          tunnel: [_ w185] -> w139
          tunnel: T6[] ["voltage", "current", "power", "speed", "measured_power", "pressure", "lsi_magnet_temp", "fisf_magnet_temp", "iir_magnet_temp"] ("Parameter") -> [_ w180]
          tunnel: [w167 w172] -> w140
          tunnel: [w167 w170] -> w130
          frame False {
            w166 = "Skip" ("software string")
            n43 = Initialize Array(w166, 6 ("维数大小")) -> (w167:string[])
          }
          frame True {
            w175 = string[] ["Inlet_Blockage_Calibration_DDM_voltage", "Inlet_Blockage_Calibration_DDM_current", "Inlet_Blockage_Calibration_DDM_power", "Inlet_Blockage_Calibration_DDM_speed", "Inlet_Blockage_Calibration_DDM_measured_power", "Inlet_Blockage_Calibration_pressure", "Inlet_Blockage_Calibration_lsi_magnet_temp", "Inlet_Blockage_Calibration_fisf_magnet_temp", "Inlet_Blockage_Calibration_iir_magnet_temp"]
            (unwired) string[] ["HL_DDM_voltage", "HL_DDM_current", "HL_DDM_power", "HL_DDM_speed", "HL_DDM_measured_power", "HL_DDM_pressure"]
            n44 = for {
              tunnel: [w202] -> w179 mode=indexing
              tunnel: [w201] -> w185
              tunnel: [w197] -> w182 mode=indexing
              tunnel: w180 -> [w199] mode=indexing
              shift-right: [w203] -> w194
              shift-left: w195 -> [w204]
              n45 = Build Array(w199) -> (w198:T6[])
              n46 = call "get_parameter.vi"("Parameter"=w198, "daemon reference in"=w204) -> ("error out"=w201:errorcluster, "response"=w202:string, "values"=w200:dbl[], "daemon reference out"=w203:refnum<k5>)  [unwired: 5 in, 1 out]
              n47 = Index Array(array=w200) -> (element=w197:dbl)  [unwired: 1 in]
            }
            n48 = in-place {
              w209 = 1000.0
              n49 = in-place-array #1(w182, 3, 5) -> (w208:dbl, w205:dbl)
              n50 = Divide(x=w208, y=w209) -> (x/y=w207:dbl)
              n51 = Divide(x=w205, y=w209) -> (x/y=w206:dbl)
              n52 = in-place-array #1(w207, w206) -> (w181:dbl[])  [unwired: 2 out]
            }
            n53 = Array To Spreadsheet String(delimiter (Tab)=",", array=w179, 3:"" ("format string")) -> (spreadsheet string=w176:string)
            n54 = Number To Fractional String(number=w181) -> (F-format string=w172:string[])  [unwired: 3 in]
            n55 = Interleave 1D Arrays(w175, w172) -> (w189:string[])
            n56 = Array To Spreadsheet String(delimiter (Tab)=";" ("格式字符串"), array=w189, 3:"" ("格式字符串")) -> (spreadsheet string=w186:string)
            n57 = Build Array (concatenate)(w191, w175) -> (w192:string[])
            n58 = Build Array (concatenate)(w176, w172) -> (w190:string[])
            n59 = for {
              tunnel: w196 -> [w216]
              tunnel: w190 -> [w214] mode=indexing
              tunnel: w192 -> [w213] mode=indexing
              tunnel: [w212] -> w193 mode=indexing
              tunnel: [w210] -> w171 mode=indexing
              w221 = "UIdisplay" ("Process (\"\" - local)")
              n60 = call "Select_Table_Vaule.vi"("Boolean"=TRUE, "Vaule"=w214, "Action"=w213, "Table"=w216) -> ("Result"=w212:bool, "vaule"=w215:string[])  [unwired: 6 in]
              n61 = Append True/False String(1:w212, 2:"FAIL" ("真字符串"), 3:"PASS" ("真字符串")) -> (0:w210:string)  [unwired: 1 in]
              n62 = Build Array (concatenate)(w215, w214, w210) -> (w220:string[])
              n63 = Flatten To XML(anything=w220) -> (xml string=w219:string)
              n64 = call "AMC Send Local Message.vi"("Process (\"\" - local)"=w221, "Message Value"=w219, "Message Name"=w221) -> ()  [unwired: 7 in, 2 out]
            }
            n65 = Delete From Array(array=w171, length=1 ("长度"), index=0 ("索引")) -> (array with subset deleted=w170:string[])  [unwired: 1 out]
          }
        }
        n66 = call <vilib>:"Space Constant.vi"() -> ("String"=w157:string)
        n67 = Concatenate Strings(w154, w157, w155) -> (w156:string)
        n68 = Index Array(array=w130) -> (element #1=w129:string, element #2=w128:string, element #3=w127:string, element #4=w125:string, element #5=w126:string, element #6=w124:string)  [unwired: 6 in]
        n69 = Index Array(array=w140) -> (element #1=w136:string, element #2=w135:string, element #3=w134:string, element #4=w133:string, element #5=w132:string, element #6=w131:string)  [unwired: 6 in]
        n70 = Bundle By Name(cluster=w141, "daemon reference"=w138, "Inlet Blockage Calibration.Inlet Blockage Calibration - DDM Parameter - Voltage"=w136, "Inlet Blockage Calibration.Inlet Blockage Calibration - DDM Parameter - Current"=w135, "Inlet Blockage Calibration.Inlet Blockage Calibration - DDM Parameter - Power"=w134, "Inlet Blockage Calibration.Inlet Blockage Calibration - DDM Parameter - Measured Power"=w132, "Inlet Blockage Calibration.Inlet Blockage Calibration - DDM Parameter - Speed"=w133, "Inlet Blockage Calibration.Inlet Blockage Calibration - DDM Parameter - Pressure"=w131, "Inlet Blockage Calibration_Status.Inlet Blockage Calibration - DDM Parameter - Voltage"=w129, "Inlet Blockage Calibration_Status.Inlet Blockage Calibration - DDM Parameter - Current"=w128, "Inlet Blockage Calibration_Status.Inlet Blockage Calibration - DDM Parameter - Power"=w127, "Inlet Blockage Calibration_Status.Inlet Blockage Calibration - DDM Parameter - Measured Power"=w126, "Inlet Blockage Calibration_Status.Inlet Blockage Calibration - DDM Parameter - Speed"=w125, "Inlet Blockage Calibration_Status.Inlet Blockage Calibration - DDM Parameter - Pressure"=w124) -> (w137:T1)
        n71 = Delete From Array(array=w148, length=1 ("长度"), index=0 ("索引")) -> (array with subset deleted=w147:bool[])  [unwired: 1 out]
        n72 = call "LogStatus.vi"("error in (no error)"=w139, "last message"=w161, "message"=w156) -> ("error  out"=w162:errorcluster)  [unwired: 8 in]
        n73 = Bundle By Name(cluster=w159, "Task_Detect_Calib.Inlet_Blockage_Calibration.DDM_Parameter"=w149, "Task_Detect_Calib.Inlet_Blockage_Calibration.DDM_Parameter_status"=w147) -> (w158:T3)
        n74 = case shown="Error" w139 {
          tunnel: [_ TRUE] -> w144
          tunnel: [_ "Error"] -> w143
          frame No Error {
          }
          frame Error {
          }
        }
      }
      frame "Inlet_Blockage_Calibration_Get_and_check_tester_Parameter" {
        n75 = Unbundle By Name(w255) -> ("Task_Detect_Calib.Inlet_Blockage_Calibration.DDM_Parameter"=w246:dbl[])
        n76 = Unbundle By Name(w244) -> ("Table"=w245:string[][])
        n77 = call "Select_Table_Vaule Enable_Disable.vi"("Action"=w260, "Table"=w245) -> ("Enable"=w259:bool)  [unwired: 8 in, 1 out]
        n78 = case shown="False" w259 {
          tunnel: [w269 w280] -> w261
          tunnel: w260 -> [_ w286]
          tunnel: w245 -> [_ w289]
          tunnel: [_ w279] -> w258
          tunnel: [_ w288] -> w250
          tunnel: w246 -> [_ w278]
          tunnel: [w270 w274] -> w243
          tunnel: [w270 w272] -> w226
          frame False {
            w269 = "Skip" ("software string")
            n79 = Initialize Array(w269, 4 ("维数大小")) -> (w270:string[])
          }
          frame True {
            w277 = string[] ["Inlet_Blockage_Calibration_Tester_Voltage", "Inlet_Blockage_Calibration_Tester_Current", "Inlet_Blockage_Calibration_Tester_Power", "Inlet_Blockage_Calibration_DDM_Real_Power"]
            n80 = call "Task_Detect_Calibration_Calculate_Tester_Parameter.vi"("DDM Parameter"=w278) -> ("Calculate Tester Parameter"=w279:dbl[])  [unwired: 10 in]
            n81 = Number To Fractional String(number=w279) -> (F-format string=w274:string[])  [unwired: 3 in]
            n82 = Interleave 1D Arrays(w277, w274) -> (w283:string[])
            n83 = Array To Spreadsheet String(delimiter (Tab)=";" ("格式字符串"), array=w283, 3:"" ("格式字符串")) -> (spreadsheet string=w280:string)
            n84 = Build Array (concatenate)(w286, w277) -> (w287:string[])
            n85 = Build Array (concatenate)("", w274) -> (w285:string[])
            n86 = for {
              tunnel: w289 -> [w295]
              tunnel: w285 -> [w293] mode=indexing
              tunnel: w287 -> [w292] mode=indexing
              tunnel: [w291] -> w288 mode=indexing
              tunnel: [w290] -> w273 mode=indexing
              w300 = "UIdisplay" ("Process (\"\" - local)")
              n87 = call "Select_Table_Vaule.vi"("Vaule"=w293, "Action"=w292, "Table"=w295) -> ("Result"=w291:bool, "vaule"=w294:string[])  [unwired: 7 in]
              n88 = Append True/False String(1:w291, 2:"FAIL" ("真字符串"), 3:"PASS" ("真字符串")) -> (0:w290:string)  [unwired: 1 in]
              n89 = Build Array (concatenate)(w294, w293, w290) -> (w299:string[])
              n90 = Flatten To XML(anything=w299) -> (xml string=w298:string)
              n91 = call "AMC Send Local Message.vi"("Process (\"\" - local)"=w300, "Message Value"=w298, "Message Name"=w300) -> ()  [unwired: 7 in, 2 out]
            }
            n92 = Delete From Array(array=w273, length=1 ("长度"), index=0 ("索引")) -> (array with subset deleted=w272:string[])  [unwired: 1 out]
          }
        }
        n93 = call <vilib>:"Space Constant.vi"() -> ("String"=w263:string)
        n94 = Unbundle By Name(w233) -> ("MES bool"=w237:refnum<vi>)
        n95 = Concatenate Strings(w260, w263, w261) -> (w262:string)
        n96 = call "HD_Config.vi"("Step"=enum16{"Initial", "Write", "Read"}."Read") -> ("HD Config out"=w238:T5)  [unwired: 9 in, 1 out]
        n97 = Unbundle By Name(w238) -> ("Fail_resume_mode"=w236:bool)
        n98 = property class="Bool (严格)"(reference=w237) -> ("Value"=w235:bool)  [unwired: 1 in, 2 out]
        n99 = Not(x=w235) -> (.not. x?=w234:bool)
        n100 = Or(x=w236, y=w234) -> (x .or. y?=w239:bool)
        n101 = Index Array(array=w226) -> (element #1=w225:string, element #2=w224:string, element #3=w223:string, element #4=w222:string)  [unwired: 4 in]
        n102 = Index Array(array=w243) -> (element #1=w230:string, element #2=w229:string, element #3=w228:string, element #4=w227:string)  [unwired: 4 in]
        n103 = Unbundle By Name(w255) -> ("Task_Detect_Calib.Inlet_Blockage_Calibration.DDM_Parameter_status"=w254:bool[])
        n104 = Bundle By Name(cluster=w244, "Inlet Blockage Calibration.Inlet Blockage Calibration - Tester Parameter - Voltage"=w230, "Inlet Blockage Calibration.Inlet Blockage Calibration - Tester Parameter - Current"=w229, "Inlet Blockage Calibration.Inlet Blockage Calibration - Tester Parameter - Power"=w228, "Inlet Blockage Calibration.Inlet Blockage Calibration - DDM Real Power"=w227, "Inlet Blockage Calibration_Status.Inlet Blockage Calibration - Tester Parameter - Voltage"=w225, "Inlet Blockage Calibration_Status.Inlet Blockage Calibration - Tester Parameter - Current"=w224, "Inlet Blockage Calibration_Status.Inlet Blockage Calibration - Tester Parameter - Power"=w223, "Inlet Blockage Calibration_Status.Inlet Blockage Calibration - DDM Real Power"=w222) -> (w242:T1)
        n105 = Delete From Array(array=w250, length=1 ("长度"), index=0 ("索引")) -> (array with subset deleted=w249:bool[])  [unwired: 1 out]
        n106 = Build Array (concatenate)(w254, w249) -> (w253:bool[])
        n107 = And Array Elements(Boolean array=w253) -> (logical AND=w232:bool)
        n108 = Select(t=TRUE, s=w239, f=w232) -> (s? t:f=w231:bool)
        n109 = call "LogStatus.vi"("error in (no error)"=w267, "last message"=w265, "message"=w262) -> ("error  out"=w266:errorcluster)  [unwired: 8 in]
        n110 = Bundle By Name(cluster=w255, "Task_Detect_Calib.Inlet_Blockage_Calibration.Get_Tester_Parameter"=w258, "Task_Detect_Calib.Inlet_Blockage_Calibration.Get_Tester_Parameter_status"=w249) -> (w264:T3)
        n111 = Not(x=w231) -> (.not. x?=w252:bool)
        n112 = Select(t="Inlet_Blockage_Calibration_Calibrate_Inlet_Blockage", s=w231, f="Finalization_NG_unit") -> (s? t:f=w251:string)
      }
      frame "Inlet_Blockage_Calibration_Calibrate_Inlet_Blockage" {
        w307 = "HH_Motor_Stop"
        n113 = Unbundle By Name(w304) -> ("Table"=w310:string[][], "daemon reference"=w316:refnum<k5>, "Config"=w309:string[][])
        n114 = call "Select_Table_Vaule Enable_Disable.vi"("Action"=w311, "Table"=w310) -> ("Enable"=w312:bool)  [unwired: 8 in, 1 out]
        n115 = case shown="True" w312 {
          tunnel: w316 -> [w323 w331]
          tunnel: [TRUE w332] -> _
          tunnel: [w323 w329] -> w302
          tunnel: ["" ("response") w328] -> w313
          tunnel: w311 -> [_ w335]
          tunnel: w310 -> [_ w334]
          tunnel: w309 -> [_ _]
          tunnel: [_ w328] -> _
          tunnel: [_ w326] -> w301
          tunnel: [_ w325] -> _
          frame False {
          }
          frame True {
            w340 = "UIdisplay" ("Process (\"\" - local)")
            n116 = call "set_calibration.vi"("values"=dbl[] [0.0], "calibration"=T7[] ["eol_inlet_blockage"], "daemon reference in"=w331) -> ("error out"=w326:errorcluster, "response"=w328:string, "daemon reference out"=w329:refnum<k5>)  [unwired: 5 in, 1 out]
            n117 = call "Select_Table_Vaule.vi"("Vaule"=w328, "Action"=w335, "Table"=w334) -> ("Result"=w332:bool, "vaule"=w333:string[])  [unwired: 7 in]
            n118 = call "时间延迟"("error in (no error)"=w326) -> ()  [unwired: 10 in, 1 out]
            n119 = Append True/False String(1:w332, 2:"FAIL" ("真字符串"), 3:"PASS" ("真字符串")) -> (0:w325:string)  [unwired: 1 in]
            n120 = Build Array (concatenate)(w333, w328, w325) -> (w339:string[])
            n121 = Flatten To XML(anything=w339) -> (xml string=w338:string)
            n122 = call "AMC Send Local Message.vi"("Process (\"\" - local)"=w340, "Message Value"=w338, "Message Name"=w340) -> ()  [unwired: 7 in, 2 out]
          }
        }
        n123 = call <vilib>:"Space Constant.vi"() -> ("String"=w315:string)
        n124 = Concatenate Strings(w311, w315, w313) -> (w314:string)
        n125 = Bundle By Name(cluster=w304, "daemon reference"=w302) -> (w303:T1)
        n126 = call "LogStatus.vi"("error in (no error)"=w301, "last message"=w317, "message"=w314) -> ("error  out"=w318:errorcluster)  [unwired: 8 in]
        n127 = case shown="Error" w301 {
          tunnel: [w320 "Error"] -> w308
          tunnel: w307 -> [w320 _]
          frame No Error {
          }
          frame Error {
          }
        }
      }
    }
    n128 = call "6-AlarmStatus.vi"("Step"=enum16{"Initial", "Write", "Read"}."Read") -> ("AlarmValue Out"=w18:bool[])  [unwired: 9 in, 1 out]
    n129 = call "Stop.vi"("Step"=enum16{"Initial", "Write", "Read"}."Read") -> ("Stop Out"=w26:bool)  [unwired: 9 in, 1 out]
    n130 = call "Exit.vi"("Step"=enum16{"Initial", "Write", "Read"}."Read" ("step")) -> ("Exit Out"=w25:bool)  [unwired: 9 in, 1 out]
    n131 = Or Array Elements(Boolean array=w18) -> (logical OR=w17:bool)
    n132 = Compound Arithmetic op=OR(w24, w26, w25, w17) -> (w23:bool)
    n133 = call "AMC Run Step.vi"("Message Queue In"=w44, "Message Name"=w32, "Message Value"=w30, "error in (no error)"=w39, "Mli/Sig"=FALSE) -> ("Message Queue Out"=w43:T4, "error out"=w38:errorcluster)  [unwired: 13 in]
  }
  "Message Queue Out" <- w6
  "error out" <- w5
  "Data" <- w10
  "Flow" <- w7
  "Data out" <- w1
